vi "triangle_demo.vi"() -> ()   [LabVIEW 2014]
panel:
  out "‰sŠp":bool
  out "space":dbl
  in  "width":dbl
  in  "height":dbl
  # "height"
  # "width"
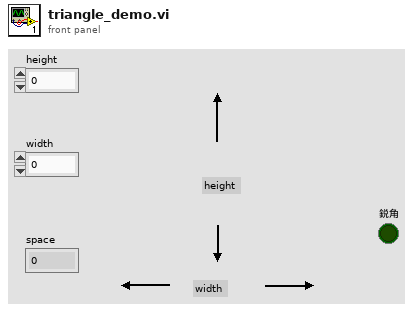
[diagram p1: front panel]
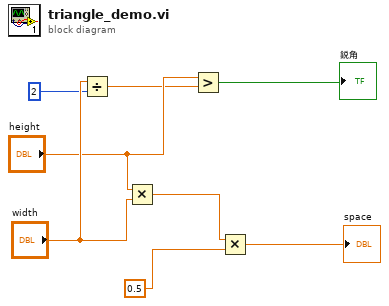
[diagram p0: block diagram]
diagram:
  n1 = Divide(x="width", y=2) -> (x/y=w2:dbl)
  n2 = Multiply(x="height", y="width") -> (x*y=w8:dbl)
  n3 = Greater?(x="height", y=w2) -> (0:→"‰sŠp":bool)
  n4 = Multiply(x=w8, y=0.5) -> (x*y=→"space":dbl)
